vi "Add Transfers Buffers with Children.vi"(6 "Decimation":u64, 7 "buffer descriptor":T1={"buffer type"=enum."Engine", "plugin id"=-1, "group id"=-1, "transfer id"=-1, "offset"=0, "length"=-1}, 8 "error in (no error)":errorcluster, 9 "Transfer Configuration":refnum<class "Transfer Configuration.lvclass">, 10 "parent tag":string, 11 "Application Data In":T3 {"current buffer data"."channels"."configuration"."string offset" format="%d bytes"; "current buffer data"."avg bandwidth" format="%.0g bytes"}) -> (0 "error out":errorcluster, 3 "Application Data out":T3 {"current buffer data"."channels"."configuration"."string offset" format="%d bytes"; "current buffer data"."avg bandwidth" format="%.0g bytes"})   [LabVIEW 2017, in "Data Viewer.lvlib"]
uses:
  Core/VIs/Data Viewer/Source/Data Viewer.lvlib
  Main VI/Application Data.ctl
  <vilib>/NI/Memory Manager/Classes/Pointer/Pointer.lvclass
  VeriStand/Data Sharing Custom Device/Source/DSF Core.lvlibp/Classes/Configuration/Core/Framework/Framework Configuration.lvclass
  Buffer Reader/Queue Data.ctl
  Buffer Reader/Buffer Data.ctl
  VeriStand/Data Sharing Custom Device/Source/DSF Core.lvlibp/Classes/Configuration/Core/Transfer/Channel Configuration.ctl
  VeriStand/Data Sharing Custom Device/Source/DSF Core.lvlibp/Typedefs/Core Channel Configuration.ctl
  VeriStand/Data Sharing Custom Device/Source/DSF Core.lvlibp/Typedefs/DSF Data Type.ctl
  VeriStand/Data Sharing Custom Device/Source/DSF Core.lvlibp/Typedefs/DSF Settings Info.ctl
  VeriStand/Data Sharing Custom Device/Source/DSF Core.lvlibp/Typedefs/DSF Byte Order.ctl
  VeriStand/Data Sharing Custom Device/Source/DSF Core.lvlibp/Classes/Thread/Data Server/DSF Buffer Subset Descriptor.ctl
  VeriStand/Data Sharing Custom Device/Source/DSF Core.lvlibp/Typedefs/DSF Buffer Type.ctl
  Main VI/Values Channels.ctl
  VeriStand/Data Sharing Custom Device/Source/DSF Core.lvlibp/Classes/Configuration/Core/Transfer/Transfer Configuration.lvclass
  Tree Item Type.ctl
  VeriStand/Data Sharing Custom Device/Source/DSF Core.lvlibp
  VeriStand/Data Sharing Custom Device/Source/DSF Core.lvlibp/Classes/Configuration/Core/Channel/Channel Configuration.lvclass
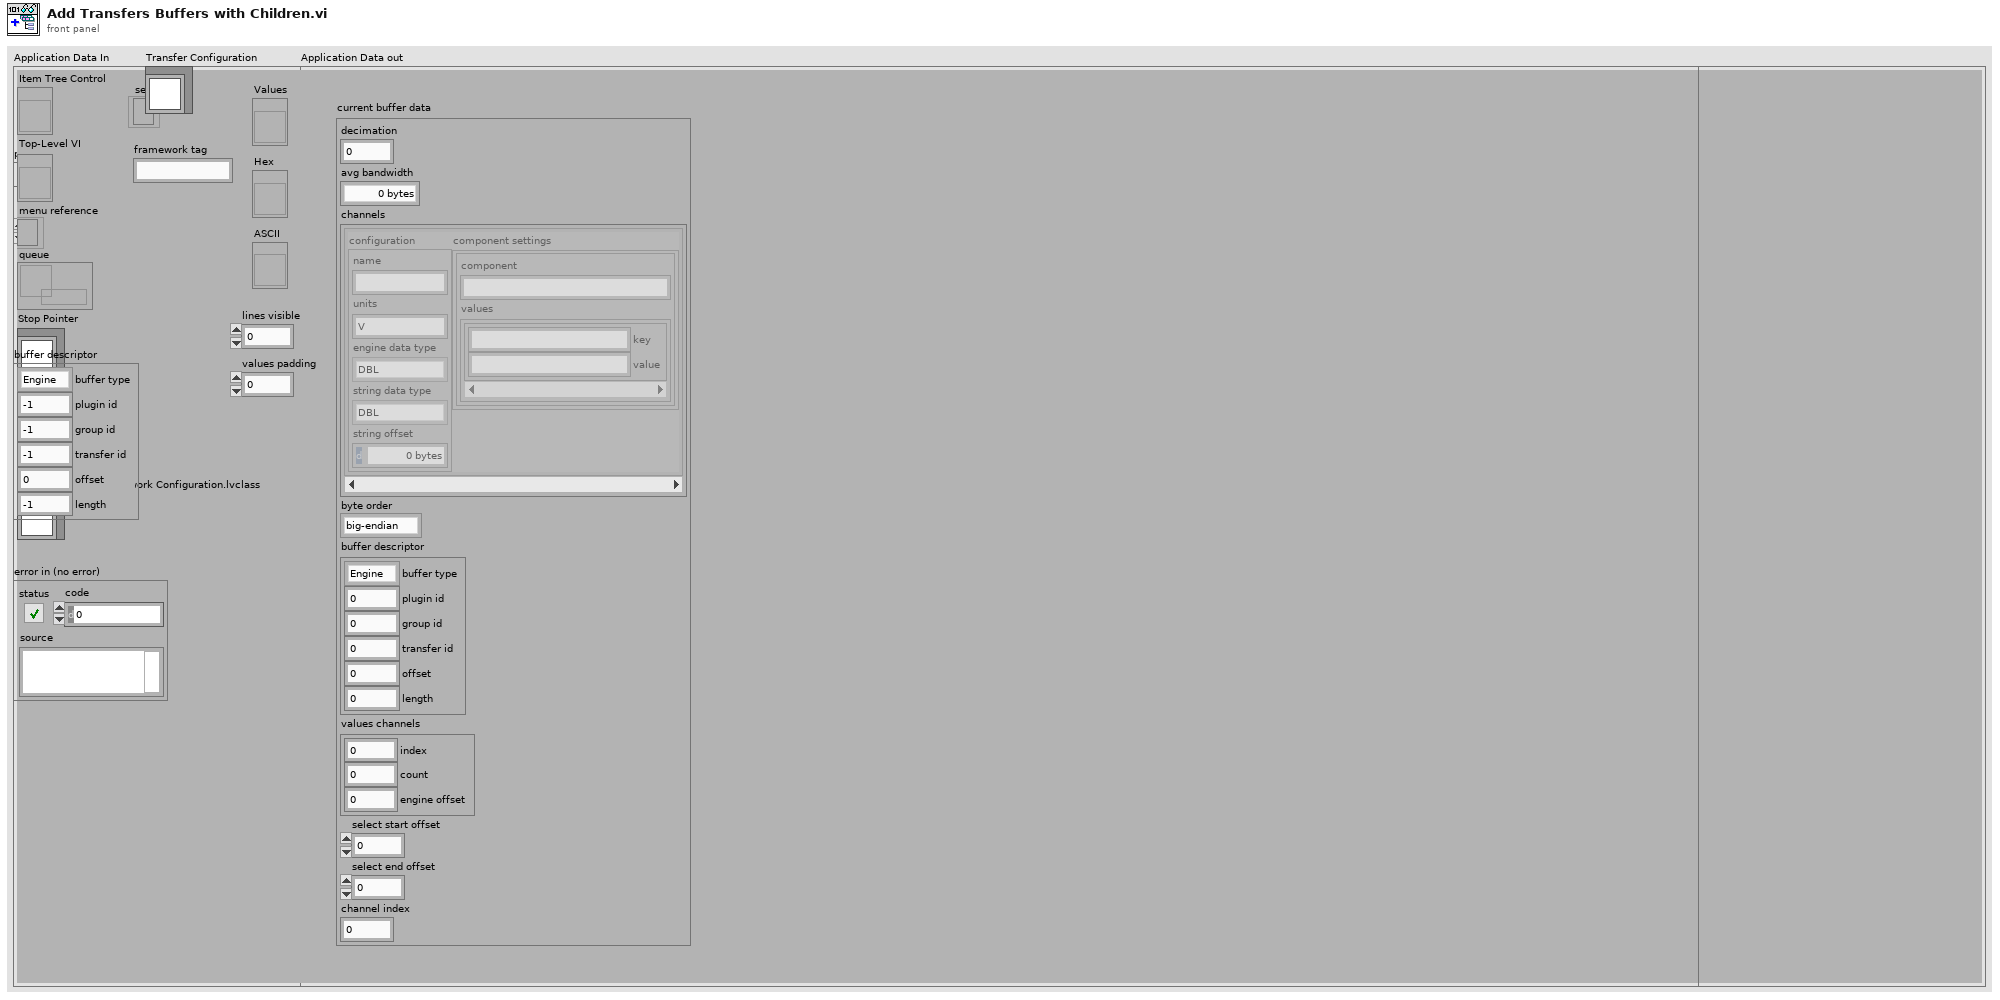
[diagram p1: front panel]
types:
  T1 = typedef "DSF Core.lvlibp/DSF Buffer Subset Descriptor.ctl" = cluster{"buffer type":T2, "plugin id":i32, "group id":i32, "transfer id":i32, "offset":u64, "length":i64}
  T2 = typedef "DSF Core.lvlibp/DSF Buffer Type.ctl" = enum16{"Engine", "String"}
  T3 = typedef "Data Viewer.lvlib/Application Data.ctl" = cluster{"Item Tree Control":refnum<vi>, "Top-Level VI":refnum<vi>, "menu reference":refnum<k9>, "queue":refnum<queue>, "Stop Pointer":refnum<class "Pointer.lvclass">, "Buffer Variant":variant, "server ID":refnum<k5>, "framework tag":string, "Values":refnum<vi>, "Hex":refnum<vi>, "ASCII":refnum<vi>, "lines visible":i32, "values padding":i32, "current buffer data":T4, "DSF Core.lvlibp:Framework Configuration.lvclass":refnum<class "Framework Configuration.lvclass">}
  T4 = typedef "Data Viewer.lvlib/Buffer Data.ctl" = cluster{"decimation":u64, "avg bandwidth":dbl, "channels":T5[], "byte order":T9, "buffer descriptor":T1, "values channels":T10, "select start offset":u64, "select end offset":u64, "channel index":i32}
  T5 = typedef "DSF Core.lvlibp/Transfer Configuration.lvclass/Channel Configuration.ctl" = cluster{"configuration":T6, "component settings":T8[]}
  T6 = typedef "DSF Core.lvlibp/Channel Configuration.lvclass/Core Channel Configuration.ctl" = cluster{"name":string, "units":string, "engine data type":T7, "string data type":T7, "string offset":u64}
  T7 = typedef "DSF Core.lvlibp/DSF Data Type.ctl" = enum8{"Bool", "SGL", "DBL", "I8", "I16", "I32", "I64", "U8", "U16", "U32", "U64"}
  T8 = typedef "DSF Core.lvlibp/DSF Settings Info.ctl" = cluster{"component":string, "values":cluster{"key":string, "value":string}[]}
  T9 = typedef "DSF Core.lvlibp/DSF Byte Order.ctl" = enum8{"big-endian", "little-endian"}
  T10 = typedef "Data Viewer.lvlib/Values Channels.ctl" = cluster{"index":i32, "count":i32, "engine offset":u64}
  T11 = typedef "Data Viewer.lvlib/Tree Item Type.ctl" = enum16{"Framework", "Plugin Group", "Plugin", "Group", "Transfer", "Buffer", "Channel"}
  T12 = typedef "Data Viewer.lvlib/Tree Item.ctl" = cluster{"Left Cell String":string, "Child Text":string[], "Child Tag":string, "Glyph Index":i32}
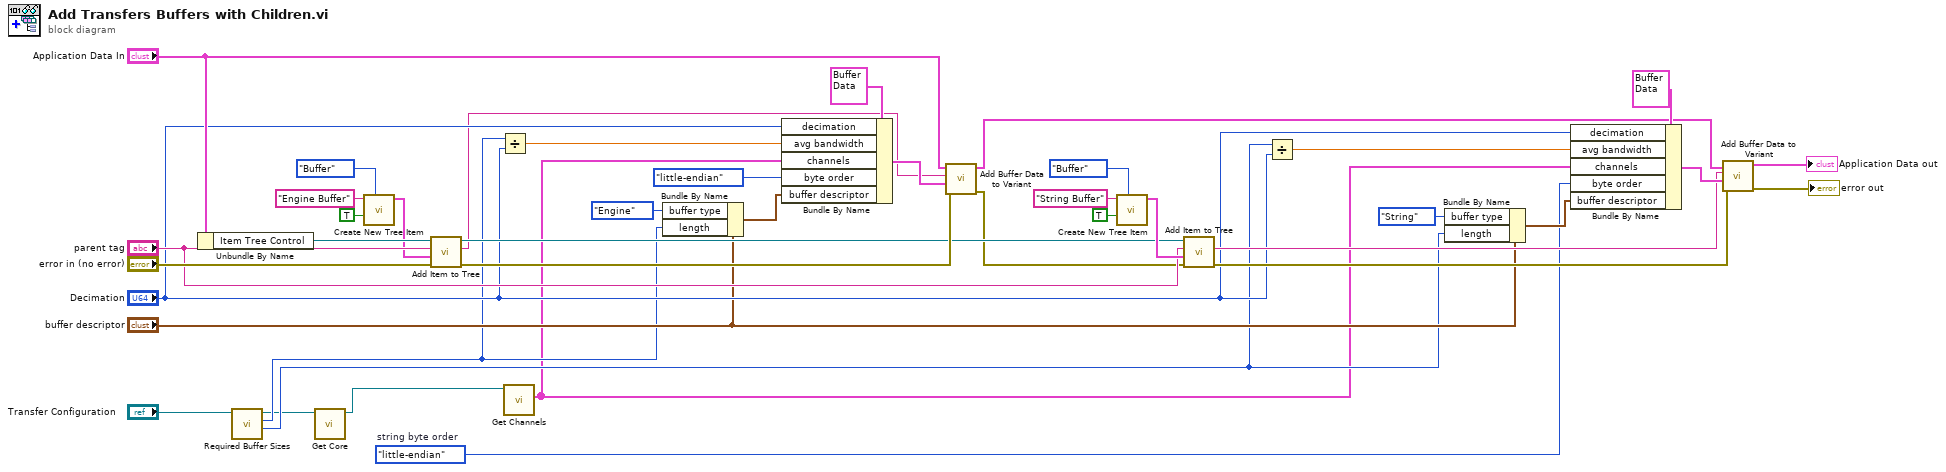
[diagram p0: block diagram]
diagram:
  w1 = DSF_Byte_Order."little-endian"  # string byte order
  n1 = Unbundle By Name("Application Data In") -> ("Item Tree Control"=w25:refnum<vi>)
  n2 = call-dynamic "Required Buffer Sizes.vi"("Transfer Configuration in"="Transfer Configuration") -> ("string size"=w7:u64, "engine size"=w6:u64, "Transfer Configuration out"=w5:refnum<class "Transfer Configuration.lvclass">)  [unwired: 7 in, 1 out]
  n3 = call "Get Core.vi"("Transfer Configuration in"=w5) -> ("Transfer Configuration out"=w4:refnum<class "Transfer Configuration.lvclass">)  [unwired: 8 in, 2 out]
  n4 = call "Create New Tree Item.vi"("Item Type"=Tree_Item_Type."Buffer", "found?"=TRUE, "Left Cell String"="Engine Buffer") -> ("Item"=w10:T12)  [unwired: 7 in, 1 out]
  n5 = call "Add Item to Tree.vi"("error in (no error)"="error in (no error)", "Item"=w10, "parent tag"="parent tag", "TreeControl in"=w25) -> ("error out"=w38:errorcluster, "new item tag"=w12:string, "TreeControl out"=w33:refnum<vi>)  [unwired: 5 in]
  n6 = Divide(x=w6, y="Decimation") -> (x/y=w18:dbl)
  n7 = call "Get Channels.vi"("Transfer Configuration in"=w4) -> ("channels"=w3:T5[])  [unwired: 8 in, 2 out]
  n8 = Bundle By Name(cluster="buffer descriptor", "buffer type"=DSF_Buffer_Type."Engine", "length"=w6) -> (w2:T1)
  n9 = Bundle By Name(cluster=T4 {"decimation"=0, "avg bandwidth"=0.0, "channels"=[], "byte order"=enum."big-endian", "buffer descriptor"={"buffer type"=enum."Engine", "plugin id"=0, "group id"=0, "transfer id"=0, "offset"=0, "length"=0}, "values channels"={"index"=0, "count"=0, "engine offset"=0}, "select start offset"=18446744073709551615, "select end offset"=0, "channel index"=-1} ("Buffer data"), "decimation"="Decimation", "avg bandwidth"=w18, "channels"=w3, "byte order"=DSF_Byte_Order."little-endian", "buffer descriptor"=w2) -> (w37:T4)
  n10 = call "Add Buffer Data to Variant.vi"("error in (no error)"=w38, "Buffer data"=w37, "tag"=w12, "Application Data In in"="Application Data In") -> ("error out"=w9:errorcluster, "Application Data In out"=w24:T3)  [unwired: 6 in]
  n11 = call "Create New Tree Item.vi"("Item Type"=Tree_Item_Type."Buffer", "found?"=TRUE, "Left Cell String"="String Buffer") -> ("Item"=w34:T12)  [unwired: 7 in, 1 out]
  n12 = call "Add Item to Tree.vi"("error in (no error)"=w9, "Item"=w34, "parent tag"="parent tag", "TreeControl in"=w33) -> ("error out"=w41:errorcluster, "new item tag"=w21:string)  [unwired: 5 in, 1 out]
  n13 = Divide(x=w7, y="Decimation") -> (x/y=w19:dbl)
  n14 = Bundle By Name(cluster="buffer descriptor", "buffer type"=DSF_Buffer_Type."String", "length"=w7) -> (w11:T1)
  n15 = Bundle By Name(cluster=T4 {"decimation"=0, "avg bandwidth"=0.0, "channels"=[], "byte order"=enum."big-endian", "buffer descriptor"={"buffer type"=enum."Engine", "plugin id"=0, "group id"=0, "transfer id"=0, "offset"=0, "length"=0}, "values channels"={"index"=0, "count"=0, "engine offset"=0}, "select start offset"=18446744073709551615, "select end offset"=0, "channel index"=-1} ("Buffer data"), "decimation"="Decimation", "avg bandwidth"=w19, "channels"=w3, "byte order"=w1, "buffer descriptor"=w11) -> (w40:T4)
  n16 = call "Add Buffer Data to Variant.vi"("error in (no error)"=w41, "Buffer data"=w40, "tag"=w21, "Application Data In in"=w24) -> ("error out"=→"error out":errorcluster, "Application Data In out"=→"Application Data out":T3)  [unwired: 6 in]
